vi "Read Address.vi"(8 "error in (no error)":errorcluster, 11 "Enumeration Tree Queue Mailman in":refnum<class "Enumeration Tree Queue Mailman.lvclass">) -> (0 "error out":errorcluster, 2 "Address":i32[](array[numeric]), 3 "Enumeration Tree Queue Mailman out":refnum<class "Enumeration Tree Queue Mailman.lvclass">)   [LabVIEW 2024, in "Enumeration Tree Queue Mailman.lvclass"]
uses:
  Enumeration Tree Queue Mailman.lvclass
  Simple Tree Queue Mailman/Simple Tree Queue Mailman.lvclass
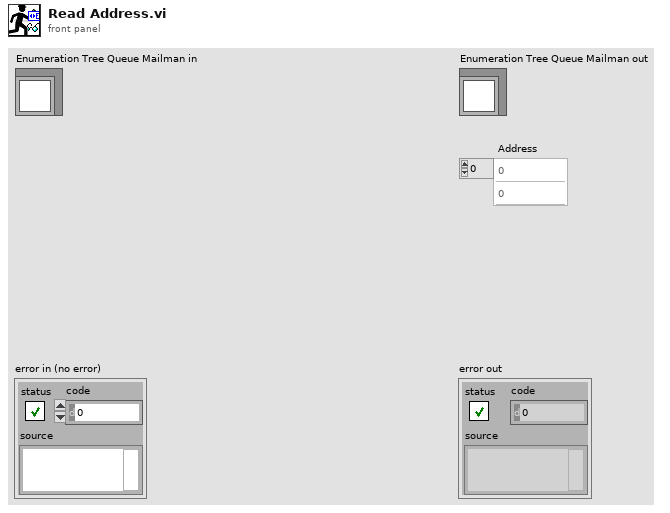
[diagram p1: front panel]
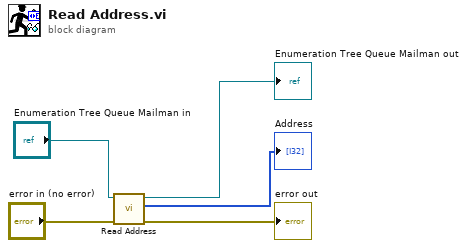
[diagram p0: block diagram]
diagram:
  n1 = call-parent "Read Address.vi"("error in (no error)"="error in (no error)", "Simple Tree Queue Mailman in"="Enumeration Tree Queue Mailman in") -> ("error out"=→"error out":errorcluster, "Address"=→"Address":i32[], "Simple Tree Queue Mailman out"=→"Enumeration Tree Queue Mailman out":refnum<class "Enumeration Tree Queue Mailman.lvclass">)  [unwired: 7 in]
